vi "Convert DST to String.vi"(5 "Initial string":string, 7 "Time":T1={"Month (Mar)"=3, "Week (2nd)"=2, "Weekday (Sun)"=0, "Hour (2)"=2} {"Hour (2)" min=0 max=23; "Weekday (Sun)" items=["Sun", "Mon", "Tue", "Wed", "Thu", "Fri", "Sat"]; "Week (2nd)" items=["1st"=1, "2nd"=2, "3rd"=3, "4th"=4, "Last"=5]; "Month (Mar)" items=["Jan"=1, "Feb"=2, "Mar"=3, "Apr"=4, "May"=5, "Jun"=6, "Jul"=7, "Aug"=8, "Sep"=9, "Oct"=10, "Nov"=11, "Dec"=12]}, 11 "error in (no error)":errorcluster) -> (6 "Resulting string":string, 15 "error out":errorcluster)   [LabVIEW 2020, in "Yokogawa GX Series.lvlib"]
doc: "Converts DST cluster to string and concatenate to initial string."
uses:
  <instrlib>/Yokogawa GX Series/Yokogawa GX Series.lvlib
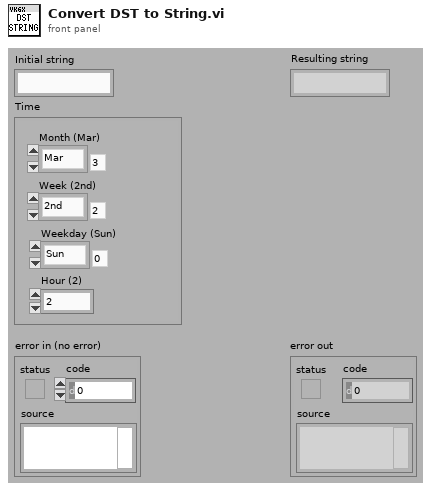
[diagram p1: front panel]
types:
  T1 = cluster{"Month (Mar)":u16, "Week (2nd)":u16, "Weekday (Sun)":u16, "Hour (2)":i32}
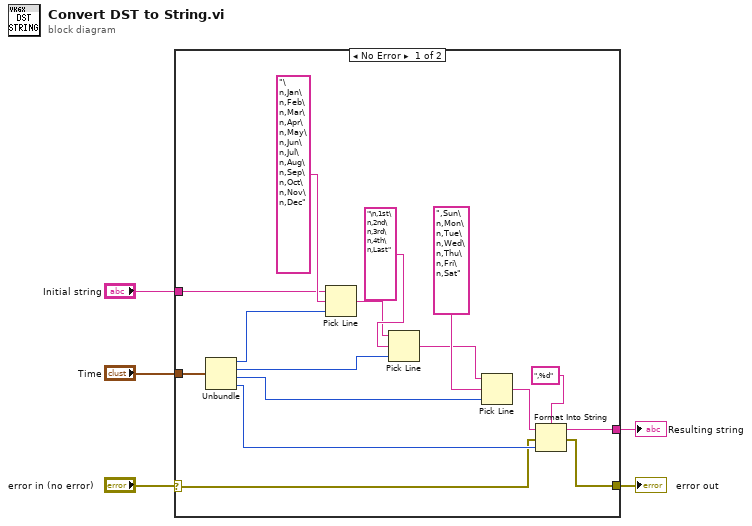
[diagram p0: block diagram]
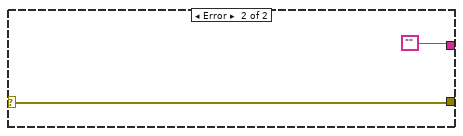
[diagram p2: hidden frame]
diagram:
  n1 = case shown="No Error" "error in (no error)" {
    selector: "error in (no error)" -> [w6 w23]
    tunnel: "Time" -> [w14 _]
    tunnel: [w9 w23] -> w4
    tunnel: [w8 ""] -> w3
    tunnel: "Initial string" -> [w7 _]
    frame No Error {
      n2 = Unbundle(w14) -> ("Month (Mar)"=w13:u16, "Week (2nd)"=w12:u16, "Weekday (Sun)"=w11:u16, "Hour (2)"=w10:i32)
      n3 = Pick Line(string ("")=w7, multi-line string="\n,Jan\n,Feb\n,Mar\n,Apr\n,May\n,Jun\n,Jul\n,Aug\n,Sep\n,Oct\n,Nov\n,Dec", line index=w13) -> (output string=w16:string)
      n4 = Pick Line(string ("")=w16, multi-line string="\n,1st\n,2nd\n,3rd\n,4th\n,Last", line index=w12) -> (output string=w18:string)
      n5 = Pick Line(string ("")=w18, multi-line string=",Sun\n,Mon\n,Tue\n,Wed\n,Thu\n,Fri\n,Sat", line index=w11) -> (output string=w20:string)
      n6 = Format Into String(format string=",%d", initial string=w20, error in=w6, w10) -> (resulting string=w8:string, error out=w9:errorcluster)
    }
    frame Error {
    }
  }
  "error out" <- w4
  "Resulting string" <- w3
